vi "coordonnées_cellule.vi"(9 "Numeric":i32, 10 "Numeric 2":i32, 11 "subset rect in":T1) -> (3 "subset rect out":T1)   [LabVIEW 2023]
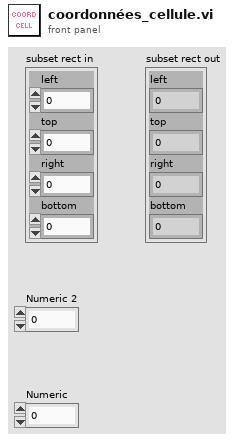
[diagram p1: front panel]
types:
  T1 = cluster{"left":i16, "top":i16, "right":i16, "bottom":i16}
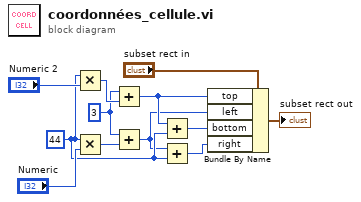
[diagram p0: block diagram]
diagram:
  w7 = 3 ("Numeric 5")
  w5 = 44 ("Numeric 3")
  n1 = Multiply(x=w5, y="Numeric 2") -> (x*y=w8:i32)
  n2 = Multiply(x=w5, y="Numeric") -> (x*y=w6:i32)
  n3 = Add(x=w7, y=w8) -> (x+y=w2:i32)
  n4 = Add(x=w7, y=w6) -> (x+y=w1:i32)
  n5 = Add(x=w2, y=w5) -> (x+y=w3:i32)
  n6 = Add(x=w1, y=w5) -> (x+y=w4:i32)
  n7 = Bundle By Name(cluster="subset rect in", "top"=w2, "left"=w1, "bottom"=w3, "right"=w4) -> (→"subset rect out":T1)
